vi "API String to 1D Array.vi"(7 "delimiter":string, 8 "error in (no error)":errorcluster, 10 "trimmed string in":string) -> (0 "error out":errorcluster, 1 "Array of Strings":string[](array[string]))   [LabVIEW 2017, in "API String Arguments Support.lvlib"]
uses:
  API String Arguments Support.lvlib
  <userlib>/_NEVSTOP/Communicable State Machine(CSM)/Communicable State Machine.lvlib
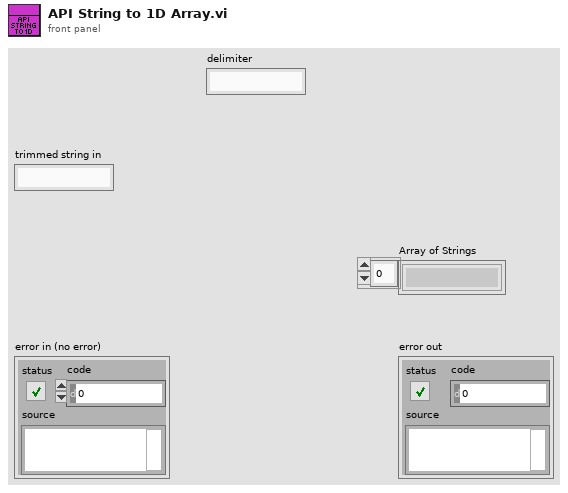
[diagram p1: front panel]
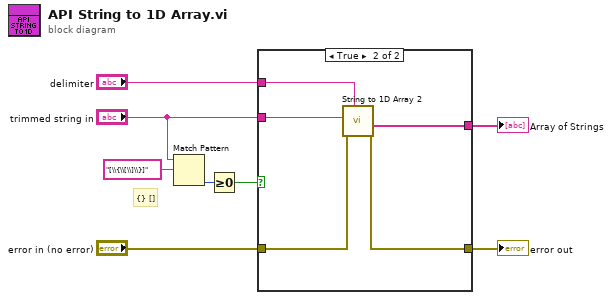
[diagram p0: block diagram]
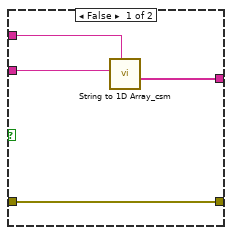
[diagram p2: hidden frame]
diagram:
  # "{} []"
  n1 = Match Pattern(string="trimmed string in", regular expression="[\\{\\[\\]\\}]") -> (offset past match=w2:i32)  [unwired: 1 in, 3 out]
  n2 = Greater Or Equal To 0?(x=w2) -> (x >= 0?=w5:bool)
  n3 = case shown="True" w5 {
    tunnel: [w12 w16] -> w1
    tunnel: "trimmed string in" -> [w11 w17]
    tunnel: "error in (no error)" -> [w10 w15]
    tunnel: [w10 w14] -> w7
    tunnel: "delimiter" -> [w9 w13]
    frame False {
      n4 = call <userlib>:"String to 1D Array_csm.vi"("delimiter (Tab)"=w9, "string"=w11) -> ("Array of Strings"=w12:string[])  [unwired: 9 in]
    }
    frame True {
      n5 = call "String to 1D Array 2.vi"("delimiter (,)"=w13, "Error in"=w15, "string"=w17) -> ("Error out"=w14:errorcluster, "Array of Strings"=w16:string[])  [unwired: 7 in]
    }
  }
  "error out" <- w7
  "Array of Strings" <- w1
